vi "AI Read Channel.vi"(1 "Samples (1)":i32=1, 2 "Channel":i32, 3 "Device":i32) -> (0 "Value":dbl format="%.3f")   [LabVIEW 2010]
uses:
  <vilib>/DAQmx/read.llb/DAQmx Read (Analog 1D DBL 1Chan NSamp).vi
  <vilib>/DAQmx/create/channels.llb/DAQmx Create Channel (AI-Voltage-Basic).vi
  <vilib>/daqmx/miscellaneous.llb/DAQmx Fill In Error Info.vi
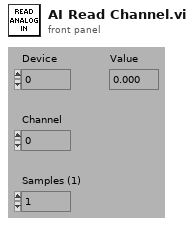
[diagram p1: front panel]
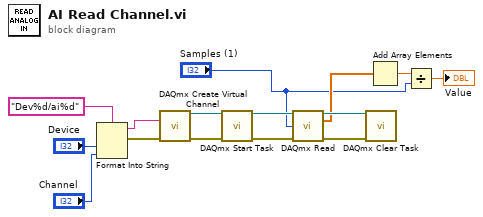
[diagram p0: block diagram]
diagram:
  n1 = Format Into String(format string="Dev%d/ai%d", "Device", "Channel") -> (resulting string=w5:string, error out=w6:errorcluster)  [unwired: 2 in]
  n2 = call-poly <vilib>:"DAQmx Create Virtual Channel.vi"("physical channels"=w5, "error in"=w6) -> ("task out"=w13:refnum<k21>, "error out"=w12:errorcluster)  [unwired: 12 in]
  n3 = call <vilib>:"DAQmx Start Task.vi"("task/channels in"=w13, "error in"=w12) -> ("task out"=w11:refnum<k21>, "error out"=w10:errorcluster)  [unwired: 12 in]
  n4 = call-poly <vilib>:"DAQmx Read.vi"("task/channels in"=w11, "number of samples per channel"="Samples (1)", "error in"=w10) -> ("task out"=w9:refnum<k21>, "data"=w4:dbl[], "error out"=w8:errorcluster)  [unwired: 10 in]
  n5 = call <vilib>:"DAQmx Clear Task.vi"("task in"=w9, "error in"=w8) -> ()  [unwired: 13 in, 1 out]
  n6 = Add Array Elements(numeric array=w4) -> (sum=w3:dbl)
  n7 = Divide(x=w3, y="Samples (1)") -> (x/y=→"Value":dbl)
